vi "Configure Digital Alarm Type.vi"(7 "Unit Address (1)":u8=1, 8 "error in (no error)":errorcluster, 9 "Alarm Type (0: No Alarm)":u8(ring) items=["No Alarm", "Positive Edge", "Negative Edge", "Edge Triggered Alarm", "High Alarm", "Low Alarm"], 10 "Alarm Number (1)":u16=1 min=1 max=8, 11 "VISA resource name":refnum<visa-resource-name>) -> (0 "error out":errorcluster, 3 "VISA resource name out":refnum<visa-resource-name>)   [LabVIEW 2014, in "Eurotherm 35xx Series.lvlib"]
doc: "This VI configure digital alarm type.\nThe type of alarm determines when it will be triggered. Examples are a high, where the input value has to be a logic '1' to set the alarm off.\n\nWarning: This VI uses Controller Configuration Mode, this interrupts working process (device will not control).\nIt is recommended that the device should be disconnected from any active process."
uses:
  <instrlib>/Eurotherm 35xx Series/Eurotherm 35xx Series.lvlib
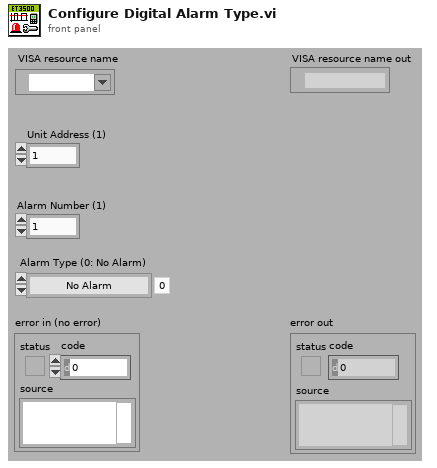
[diagram p1: front panel]
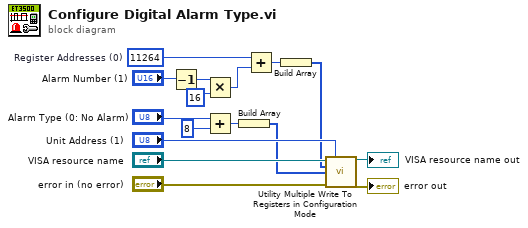
[diagram p0: block diagram]
diagram:
  w12 = 11264  # Register Addresses (0)
  n1 = Decrement(x="Alarm Number (1)") -> (x-1=w15:u16)
  n2 = Multiply(x=w15, y=u16 16) -> (x*y=w13:u16)
  n3 = Add(x="Alarm Type (0: No Alarm)", y=u8 8) -> (x+y=w3:u8)
  n4 = Build Array(w3) -> (w6:u8[])
  n5 = Add(x=w12, y=w13) -> (x+y=w5:i32)
  n6 = Build Array(w5) -> (w4:i32[])
  n7 = call <instrlib>:"Utility Multiple Write To Registers in Configuration Mode.vi"("VISA resource name"="VISA resource name", "Unit Address (1)"="Unit Address (1)", "Registers Addresses (0)"=w4, "Data (0)"=w6, "error in (no error)"="error in (no error)") -> ("VISA resource name out"=→"VISA resource name out":refnum<visa-resource-name>, "error out"=→"error out":errorcluster)  [unwired: 9 in]
